vi "Set Color by ARGB(Cluster).vi"(8 "error in (no error)":errorcluster caption="错误输入（无错误）", 11 "ARGB":T1) -> (0 "error out":errorcluster caption="错误输出", 3 "FromArgb":refnum<k24>)   [LabVIEW 2012, in "Color.lvclass"]
uses:
  Color.lvclass
  ARGB.ctl
  System.Drawing
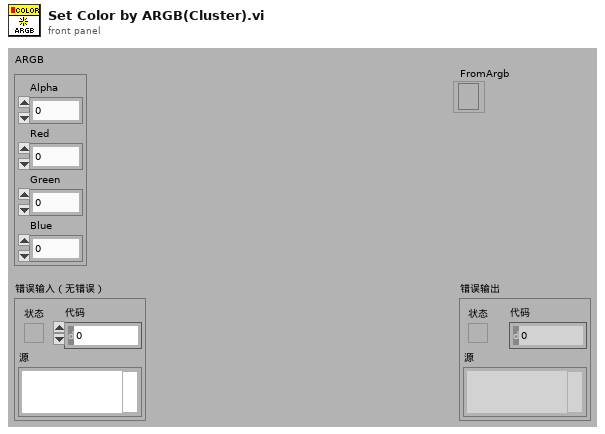
[diagram p1: front panel]
types:
  T1 = typedef "Color.lvclass/ARGB.ctl" = cluster{"Alpha":i32, "Red":i32, "Green":i32, "Blue":i32}
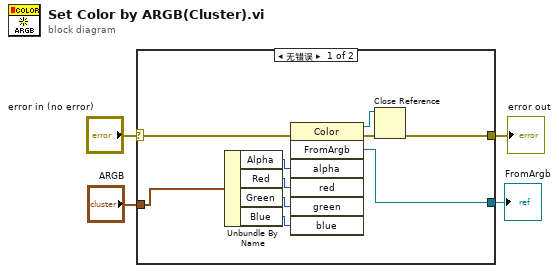
[diagram p0: block diagram]
diagram:
  n1 = case shown="无错误" "error in (no error)" {
    selector: "error in (no error)" -> [w14 w15]
    tunnel: [w13 w15] -> w3
    tunnel: "ARGB" -> [w12 _]
    tunnel: [w5 _] -> w1
    frame No Error {
      n2 = Unbundle By Name(w12) -> ("Alpha"=w11:i32, "Red"=w10:i32, "Green"=w9:i32, "Blue"=w8:i32)
      n3 = invoke class="Color" method="FromArgb"(error in=w14, "alpha"=w11, "red"=w10, "green"=w9, "blue"=w8) -> (reference out=w7:refnum<k24>, error out=w6:errorcluster, "FromArgb"=w5:refnum<k24>)  [unwired: 2 in, 4 out]
      n4 = Close Reference(reference=w7, error in (no error)=w6) -> (error out=w13:errorcluster)
    }
    frame Error {
    }
  }
  "error out" <- w3
  "FromArgb" <- w1
